vi "Set Calibration Level.vi"(8 "error in (no error)":errorcluster, 10 "DG Number":i32, 11 "CalibrationLevel":u32(ring)=2 items=["None", "CalibrateIncrement", "CalibrateOffset"]) -> (0 "error out":errorcluster)   [LabVIEW 2009, in "POLARIS BME DG.lvlib"]
doc: "long Set_CalibrationLevel(unsigned long CalibrationLevel, long DG_Number);"
uses:
  POLARIS BME DG.lvlib
  BME DLL/DelayGenerator.dll
panel:
  # "NOTICE -- YOU MUST LEAVE THIS NOTICE IN PLACE.  PER THE TERMS OF THE LICENSE BELOW, YOU MAY SUBLICENSE THIS SOFTWARE \nIN ANY WAY THAT DOES NOT CONFLICT WITH THIS LICENSE.\n\n### BSD License (http://www.opensource.org/licenses/bsd-license.php) Begin ###\n \nCopyright (c) 2011, Applied Energetics, http://www.appliedenergetics.com,\n                               Richard Schwerdtfeger, <rschwerdtfeger@appliedenergetics.com>\n\nAll rights reserved.\n\nRedistribution and use in source and binary forms, with or without modification, are permitted provided that the \nfollowing conditions are met:\n\n    * Redistributions of source code must retain the above copyright notice, this list of conditions and the following disclaimer.\n    * Redistributions in binary form must reproduce the above copyright notice, this list of conditions and the following disclaimer \n       in the documentation and/or other materials provided with the distribution.\n    * Neither the name of Richard Schwerdtfeger, Applied Energetics, Inc., nor the names of its contributors may be used to \n       endorse or promote products derived from this software without specific prior written permission.\n\nTHIS SOFTWARE IS PROVIDED BY THE COPYRIGHT HOLDERS AND CONTRIBUTORS \"AS IS\" AND ANY EXPRESS OR IMPLIED WARRANTIES, \nINCLUDING, BUT NOT LIMITED TO, THE IMPLIED WARRANTIES OF MERCHANTABILITY AND FITNESS FOR A PARTICULAR PURPOSE ARE \nDISCLAIMED. IN NO EVENT SHALL THE COPYRIGHT OWNER OR CONTRIBUTORS BE LIABLE FOR ANY DIRECT, INDIRECT, INCIDENTAL,\n SPECIAL, EXEMPLARY, OR CONSEQUENTIAL DAMAGES (INCLUDING, BUT NOT LIMITED TO, PROCUREMENT OF SUBSTITUTE GOODS OR \nSERVICES; LOSS OF USE, DATA, OR PROFITS; OR BUSINESS INTERRUPTION) HOWEVER CAUSED AND ON ANY THEORY OF LIABILITY, \nWHETHER IN CONTRACT, STRICT LIABILITY, OR TORT (INCLUDING NEGLIGENCE OR OTHERWISE) ARISING IN ANY WAY OUT OF THE USE \nOF THIS SOFTWARE, EVEN IF ADVISED OF THE POSSIBILITY OF SUCH DAMAGE.\n\n### BSD License End ###"
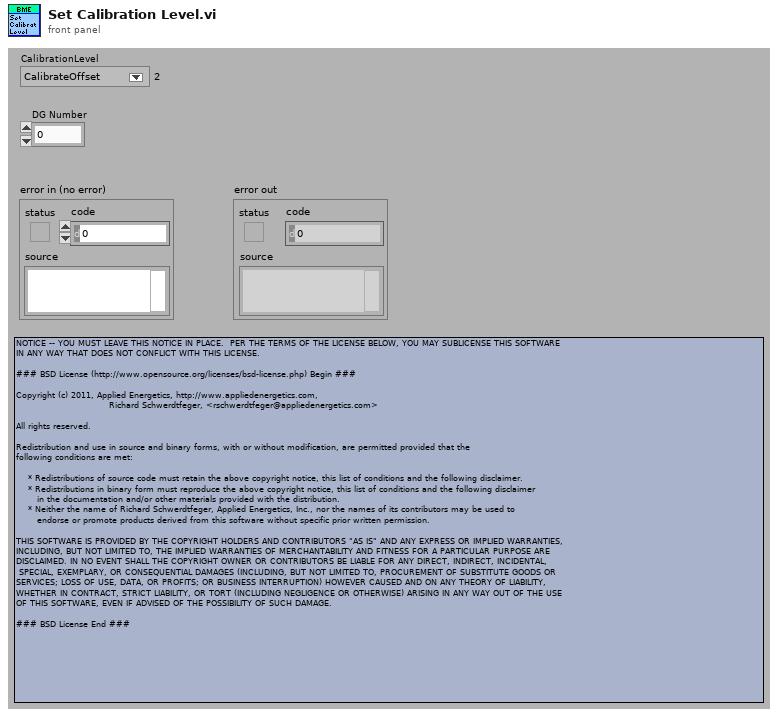
[diagram p1: front panel]
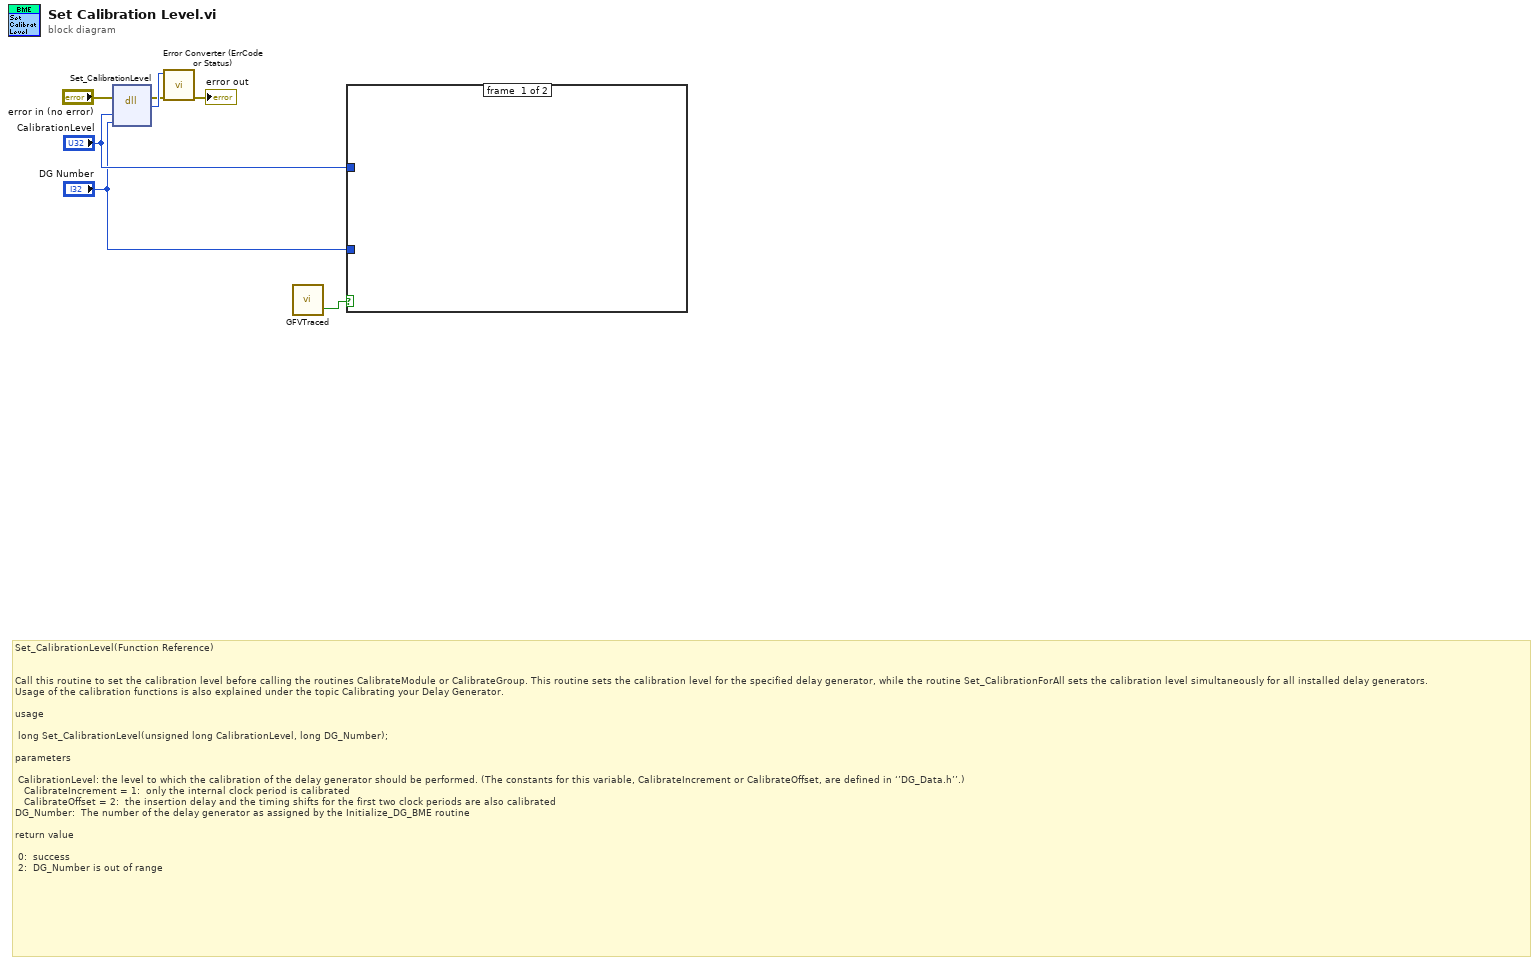
[diagram p0: block diagram]
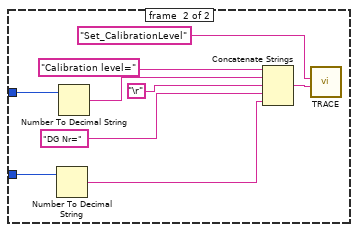
[diagram p2: hidden frame]
diagram:
  # "Set_CalibrationLevel(Function Reference)\n\n\nCall this routine to set the calibration level before calling the routines CalibrateModule or CalibrateGroup. This routine sets the calibration level for the specified delay generator, while the routine Set_CalibrationForAll sets the calibration level simultaneously for all installed delay generators.\nUsage of the calibration functions is also explained under the topic Calibrating your Delay Generator.\n\nusage\n\n\tlong Set_CalibrationLevel(unsigned long CalibrationLevel, long DG_Number);\n\nparameters\n\n\tCalibrationLevel:\tthe level to which the calibration of the delay generator should be performed. (The constants for this variable, CalibrateIncrement or CalibrateOffset, are defined in ‘’DG_Data.h’’.)\n\t\t\tCalibrateIncrement = 1:\t\tonly the internal clock period is calibrated\n\t\t\tCalibrateOffset = 2:\t\tthe insertion delay and the timing shifts for the first two clock periods are also calibrated\nDG_Number:\t\tThe number of the delay generator as assigned by the Initialize_DG_BME routine\n\nreturn value\n\n\t0:  success\n\t2:  DG_Number is out of range"
  n1 = dll-call lib="D:/CS Framework/LVSCC/LV2009/GPL/Projects/cs-framework/CSClass/CSPOLARIS/POLARIS BME DG/BME DLL/DelayGenerator.*" fn="Set_CalibrationLevel"(error in="error in (no error)", "CalibrationLevel"="CalibrationLevel", "DG_Number"="DG Number") -> (error out=w5:errorcluster, w7:i32)  [unwired: 4 in, 1 out]
  n2 = call "Error Converter (ErrCode or Status).vi"("error in (no error)"=w5, "error code"=w7) -> ("error out"=→"error out":errorcluster)  [unwired: 9 out]
  n3 = call "GFVTraced.vi"() -> ("traced?"=w3:bool)  [unwired: 2 in]
  n4 = case shown="True" w3 {
    tunnel: "CalibrationLevel" -> [_ w10]
    tunnel: "DG Number" -> [_ w8]
    frame #0 {
    }
    frame #1 {
      n5 = Number To Decimal String(number=w8) -> (decimal integer string=w9:string)  [unwired: 1 in]
      n6 = Number To Decimal String(number=w10) -> (decimal integer string=w14:string)  [unwired: 1 in]
      n7 = Concatenate Strings("Calibration level=", w14, "\r", "DG Nr=", w9) -> (w11:string)
      n8 = call "TRACE.vi"("Parameter String"=w11, "Function"="Set_CalibrationLevel") -> ()  [unwired: 10 in]
    }
  }
